vi "D1-b_Tests.vi"   [LabVIEW 2017]
uses:
  OOP/Elf/Elf.lvclass/Elf.ctl
  <vilib>/addons/_JKI Toolkits/Caraya/classes/Assert/Assert Equal Value_Variant.vi
  OOP/Elf/Elf.lvclass
  <vilib>/addons/_JKI Toolkits/Caraya/classes/Test/Test.lvclass
  <vilib>/addons/_JKI Toolkits/Caraya/classes/Assert/Assert.lvclass
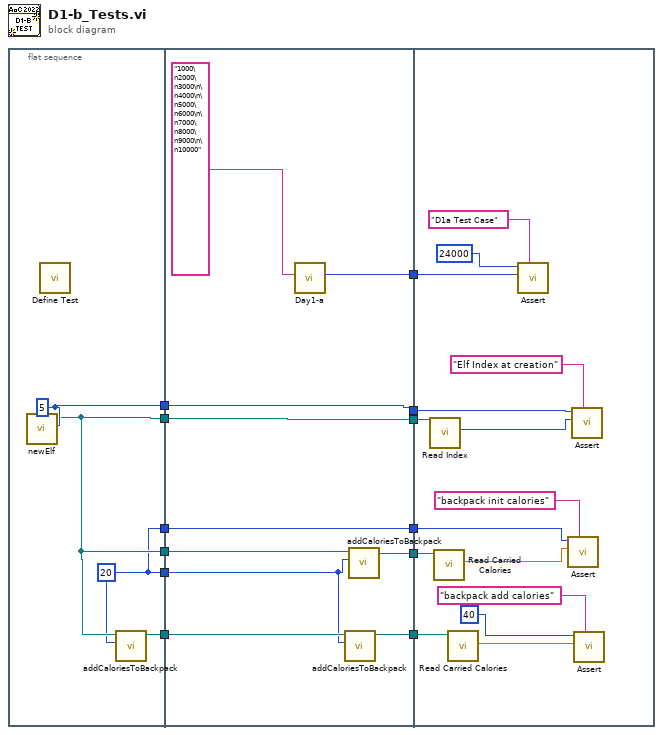
[diagram p0: block diagram]
diagram:
  n1 = flat-sequence {
    tunnel: [w16] -> w9
    tunnel: [w15] -> w8
    tunnel: [w15] -> w7
    tunnel: [w14] -> w5
    tunnel: [w14] -> w3
    tunnel: [w13] -> w2
    tunnel: [w25] -> w12
    tunnel: [w23] -> w11
    tunnel: [w24] -> w10
    tunnel: w9 -> [w24]
    tunnel: w8 -> [w23]
    tunnel: w7 -> [w22]
    tunnel: [w21] -> w6
    tunnel: w5 -> [w18]
    tunnel: [w20] -> w4
    tunnel: w3 -> [w20]
    tunnel: w2 -> [w19]
    tunnel: [w17] -> w1
    tunnel: w12 -> [w41]
    tunnel: w11 -> [w37]
    tunnel: w10 -> [w35]
    tunnel: w6 -> [w34]
    tunnel: w4 -> [w32]
    tunnel: w1 -> [w30]
    frame #0 {
      w14 = 20 ("Calories")
      w16 = 5 ("Index")
      n2 = call "newElf.vi"("Index"=w16) -> ("Elf out"=w15:refnum<class "Elf.lvclass">)  [unwired: 9 in, 1 out]
      n3 = call <vilib>:"Define Test.vi"() -> ()  [unwired: 11 in, 1 out]
      n4 = call-dynamic "addCaloriesToBackpack.vi"("Calories"=w14, "Elf in"=w15) -> ("Elf out"=w13:refnum<class "Elf.lvclass">)  [unwired: 8 in, 1 out]
    }
    frame #1 {
      n5 = call "Day1-a.vi"("Input"="1000\n2000\n3000\n\n4000\n\n5000\n6000\n\n7000\n8000\n9000\n\n10000") -> ("Output"=w25:i32)  [unwired: 10 in]
      n6 = call-dynamic "addCaloriesToBackpack.vi"("Calories"=w18, "Elf in"=w19) -> ("Elf out"=w17:refnum<class "Elf.lvclass">)  [unwired: 8 in, 1 out]
      n7 = call-dynamic "addCaloriesToBackpack.vi"("Calories"=w18, "Elf in"=w22) -> ("Elf out"=w21:refnum<class "Elf.lvclass">)  [unwired: 8 in, 1 out]
    }
    frame #2 {
      n8 = call "Read Index.vi"("Elf in"=w37) -> ("Index"=w36:i32)  [unwired: 8 in, 2 out]
      n9 = call "Read Carried Calories.vi"("Elf in"=w34) -> ("Carried Calories"=w31:dbl)  [unwired: 8 in, 2 out]
      n10 = call "Read Carried Calories.vi"("Elf in"=w30) -> ("Carried Calories"=w27:dbl)  [unwired: 8 in, 2 out]
      n11 = call-poly <vilib>:"Assert.vi"("Label"="D1a Test Case", "Y"=w41, "X"=24000 ("Output")) -> ()  [unwired: 8 in, 1 out]
      n12 = call-poly <vilib>:"Assert.vi"("Label"="backpack init calories", "Y"=w31, "X"=w32) -> ()  [unwired: 8 in, 1 out]
      n13 = call-poly <vilib>:"Assert.vi"("Label"="Elf Index at creation", "Y"=w36, "X"=w35) -> ()  [unwired: 8 in, 1 out]
      n14 = call-poly <vilib>:"Assert.vi"("Label"="backpack add calories", "Y"=w27, "X"=40 ("Calories")) -> ()  [unwired: 8 in, 1 out]
    }
  }
